vi "Load Settings from XML.vi"(8 "error in (no error)":errorcluster, 11 "Settings in":T1={"Acquisition Settings"={"AI"={"task name"="", "task_ref"="", "physical channels"="Dev1/ai0:7", "channels config"={"input terminal configuration"=0, "minimum value"=-5.0, "maximum value"=5.0}, "rate"=1000.0}, "conversions"={"ai0"={"a"=0.0, "b"=0.0}, "ai1"={"a"=0.0, "b"=0.0}, "ai2"={"a"=0.0, "b"=0.0}, "ai3"={"a"=0.0, "b"=0.0}, "ai4"={"a"=0.0, "b"=0.0}}, "compteur 0"={"task name"="CTR", "task_ref"="", "ctr"="Dev1/ctr0:3", "coeff"=4000.0}, "compteur 1"={"task name"="CTR1", "task_ref"="", "ctr"="Dev1/ctr1", "coeff"=4000.0}, "compteur 2"={"task name"="CTR2", "task_ref"="", "ctr"="Dev1/ctr2", "coeff"=4000.0}, "compteur 3"={"task name"="CTR3", "task_ref"="", "ctr"="Dev1/ctr3", "coeff"=4000.0}}, "Logging Configuration"={"Log File Base Path"=path "", "L1"={"ref"=refnum, "actif?"=FALSE, "Fsave"=0}, "L2"={"ref"=refnum, "actif?"=FALSE, "Fsave"=0}, "L3"={"ref"=refnum, "actif?"=FALSE, "Fsave"=0}, "L4"={"ref"=refnum, "actif?"=FALSE, "Fsave"=0}}, "Generation Settings"={"AO"={"task name"="AO", "task_ref"="", "physical channels"="Dev1/ao0"}, "PID"={"P"=0.0, "I"=0.0, "D"=0.0}, "conversions"={"ao0"={"a"=0.0, "b"=0.0}}, "setpoint"=0.0}, "Digital Control Configuration"={"DO"={"task name"="DO", "task_ref"="", "lines"="Dev1/port0/line2:3, Dev1/port0/line5"}}} {"Acquisition Settings"."compteur 3"."coeff" format="%0.2f"; "Acquisition Settings"."compteur 2"."coeff" format="%0.2f"; "Acquisition Settings"."compteur 1"."coeff" format="%0.2f"; "Acquisition Settings"."compteur 0"."coeff" format="%0.2f"; "Acquisition Settings"."AI"."rate" format="%0.2f"; "Acquisition Settings"."AI"."channels config"."input terminal configuration" items=["Default"=-1, "RSE"=10083, "NRSE"=10078, "Differential"=10106, "Pseudodifferential"=12529]}) -> (0 "error out":errorcluster, 3 "Settings out":T1={"Acquisition Settings"={"AI"={"task name"="", "task_ref"="", "physical channels"="Dev1/ai0:7", "channels config"={"input terminal configuration"=0, "minimum value"=-5.0, "maximum value"=5.0}, "rate"=1000.0}, "conversions"={"ai0"={"a"=0.0, "b"=0.0}, "ai1"={"a"=0.0, "b"=0.0}, "ai2"={"a"=0.0, "b"=0.0}, "ai3"={"a"=0.0, "b"=0.0}, "ai4"={"a"=0.0, "b"=0.0}}, "compteur 0"={"task name"="CTR", "task_ref"="", "ctr"="Dev1/ctr0:3", "coeff"=4000.0}, "compteur 1"={"task name"="CTR1", "task_ref"="", "ctr"="Dev1/ctr1", "coeff"=4000.0}, "compteur 2"={"task name"="CTR2", "task_ref"="", "ctr"="Dev1/ctr2", "coeff"=4000.0}, "compteur 3"={"task name"="CTR3", "task_ref"="", "ctr"="Dev1/ctr3", "coeff"=4000.0}}, "Logging Configuration"={"Log File Base Path"=path "", "L1"={"ref"=refnum, "actif?"=FALSE, "Fsave"=0}, "L2"={"ref"=refnum, "actif?"=FALSE, "Fsave"=0}, "L3"={"ref"=refnum, "actif?"=FALSE, "Fsave"=0}, "L4"={"ref"=refnum, "actif?"=FALSE, "Fsave"=0}}, "Generation Settings"={"AO"={"task name"="AO", "task_ref"="", "physical channels"="Dev1/ao0"}, "PID"={"P"=0.0, "I"=0.0, "D"=0.0}, "conversions"={"ao0"={"a"=0.0, "b"=0.0}}, "setpoint"=0.0}, "Digital Control Configuration"={"DO"={"task name"="DO", "task_ref"="", "lines"="Dev1/port0/line2:3, Dev1/port0/line5"}}} {"Acquisition Settings"."compteur 3"."coeff" format="%0.2f"; "Acquisition Settings"."compteur 2"."coeff" format="%0.2f"; "Acquisition Settings"."compteur 1"."coeff" format="%0.2f"; "Acquisition Settings"."compteur 0"."coeff" format="%0.2f"; "Acquisition Settings"."AI"."rate" format="%0.2f"; "Acquisition Settings"."AI"."channels config"."input terminal configuration" items=["Default"=-1, "RSE"=10083, "NRSE"=10078, "Differential"=10106, "Pseudodifferential"=12529]})   [LabVIEW 2014, in "PLS Settings.lvlib"]
doc: "Attempts to load previous user specified settings from an XML file.\n\nThis VI will not generate an error. If a suitable XML file can't be loaded and parsed then it will simply return the default settings."
uses:
  PLS Settings.lvlib
  Settings.ctl
  Acquisition/Hardware Configuration.ctl
  conversion.ctl
  Logging/Logging Configuration.ctl
  Generation/Hardware Configuration.ctl
  Digital Control/Hardware Configuration.ctl
  <vilib>/Utility/xml.llb/Read From XML File(string).vi
  <vilib>/Utility/xml.llb/Write to XML File(string).vi
  Acquisition/PLS Acquisition.lvlib
  Logging/PLS Logging.lvlib
  Generation/PLS Generation.lvlib
  Digital Control/PLS Digital Control.lvlib
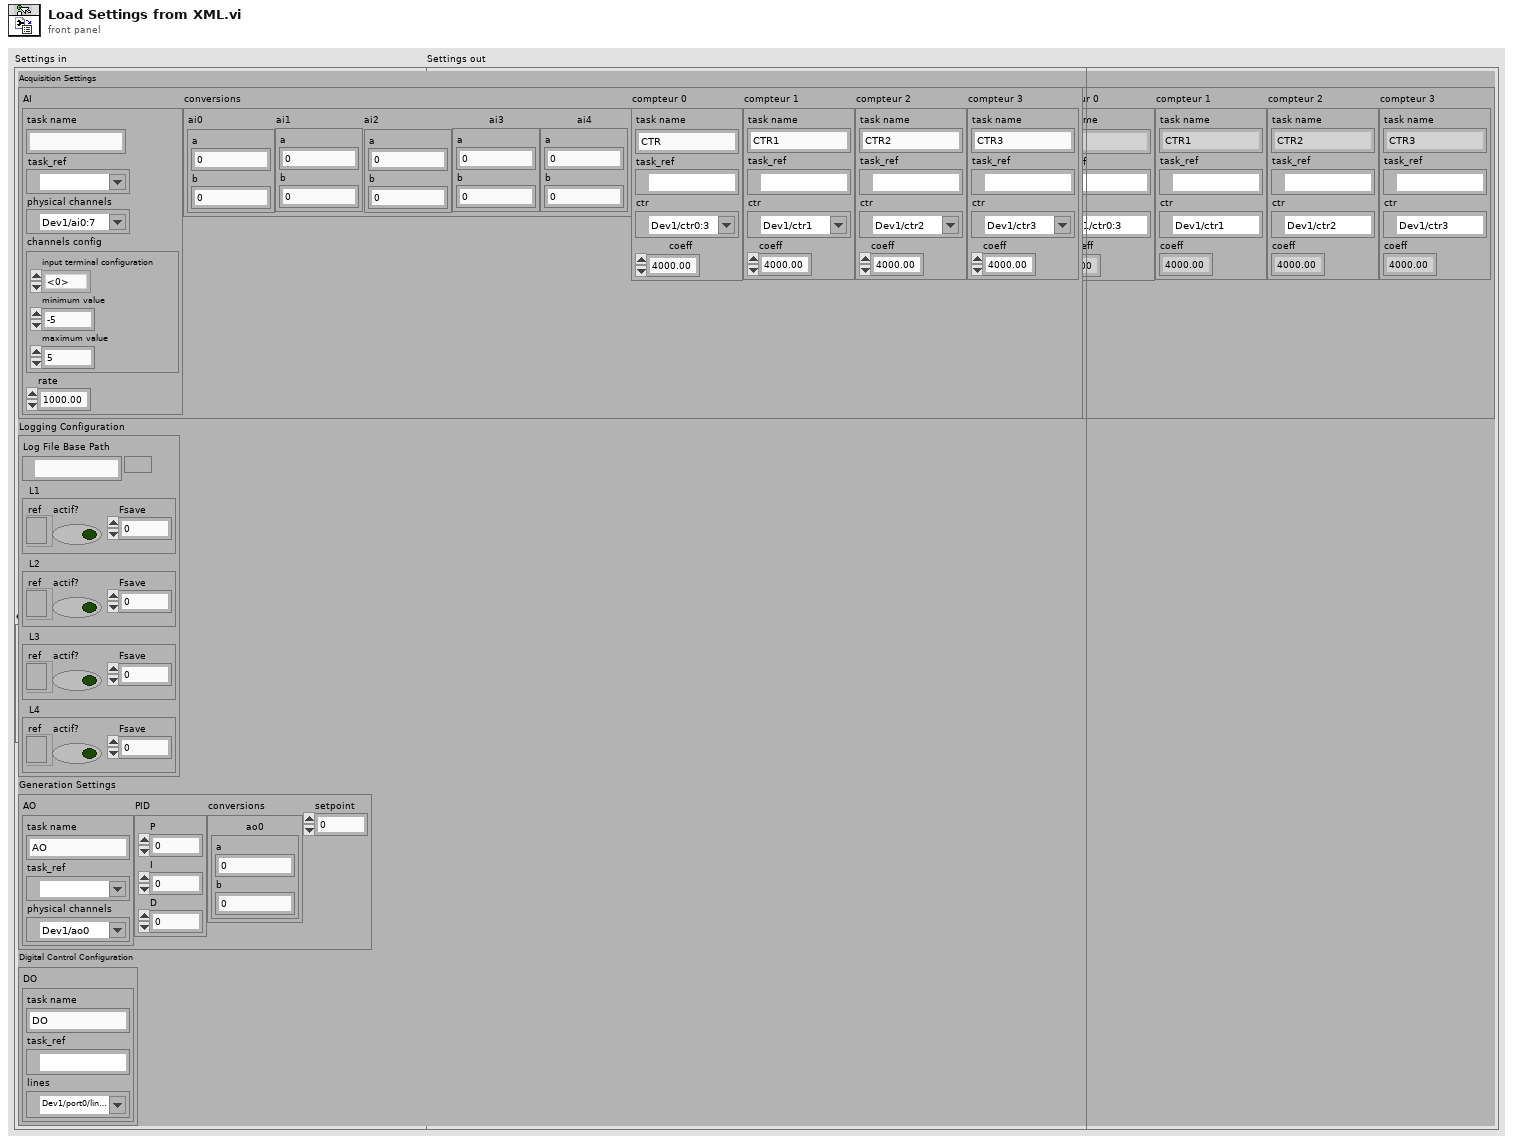
[diagram p1: front panel]
types:
  T1 = typedef "PLS Settings.lvlib/Settings.ctl" = cluster{"Acquisition Settings":T2, "Logging Configuration":T4, "Generation Settings":T5, "Digital Control Configuration":T6}
  T2 = typedef "PLS Acquisition.lvlib/Hardware Configuration.ctl" = cluster{"AI":cluster{"task name":string, "task_ref":refnum<k21>, "physical channels":tag, "channels config":cluster{"input terminal configuration":i32, "minimum value":dbl, "maximum value":dbl}, "rate":dbl}, "conversions":cluster{"ai0":T3, "ai1":T3, "ai2":T3, "ai3":T3, "ai4":T3}, "compteur 0":cluster{"task name":string, "task_ref":refnum<k21>, "ctr":tag, "coeff":dbl}, "compteur 1":cluster{"task name":string, "task_ref":refnum<k21>, "ctr":tag, "coeff":dbl}, "compteur 2":cluster{"task name":string, "task_ref":refnum<k21>, "ctr":tag, "coeff":dbl}, "compteur 3":cluster{"task name":string, "task_ref":refnum<k21>, "ctr":tag, "coeff":dbl}}
  T3 = typedef "PLS Settings.lvlib/conversion.ctl" = cluster{"a":dbl, "b":dbl}
  T4 = typedef "PLS Logging.lvlib/Logging Configuration.ctl" = cluster{"Log File Base Path":path, "L1":cluster{"ref":refnum<file>, "actif?":bool, "Fsave":i32}, "L2":cluster{"ref":refnum<file>, "actif?":bool, "Fsave":i32}, "L3":cluster{"ref":refnum<file>, "actif?":bool, "Fsave":i32}, "L4":cluster{"ref":refnum<file>, "actif?":bool, "Fsave":i32}}
  T5 = typedef "PLS Generation.lvlib/Hardware Configuration.ctl" = cluster{"AO":cluster{"task name":string, "task_ref":refnum<k21>, "physical channels":tag}, "PID":cluster{"P":dbl, "I":dbl, "D":dbl}, "conversions":cluster{"ao0":T3}, "setpoint":dbl}
  T6 = typedef "PLS Digital Control.lvlib/Hardware Configuration.ctl" = cluster{"DO":cluster{"task name":string, "task_ref":refnum<k21>, "lines":tag}}
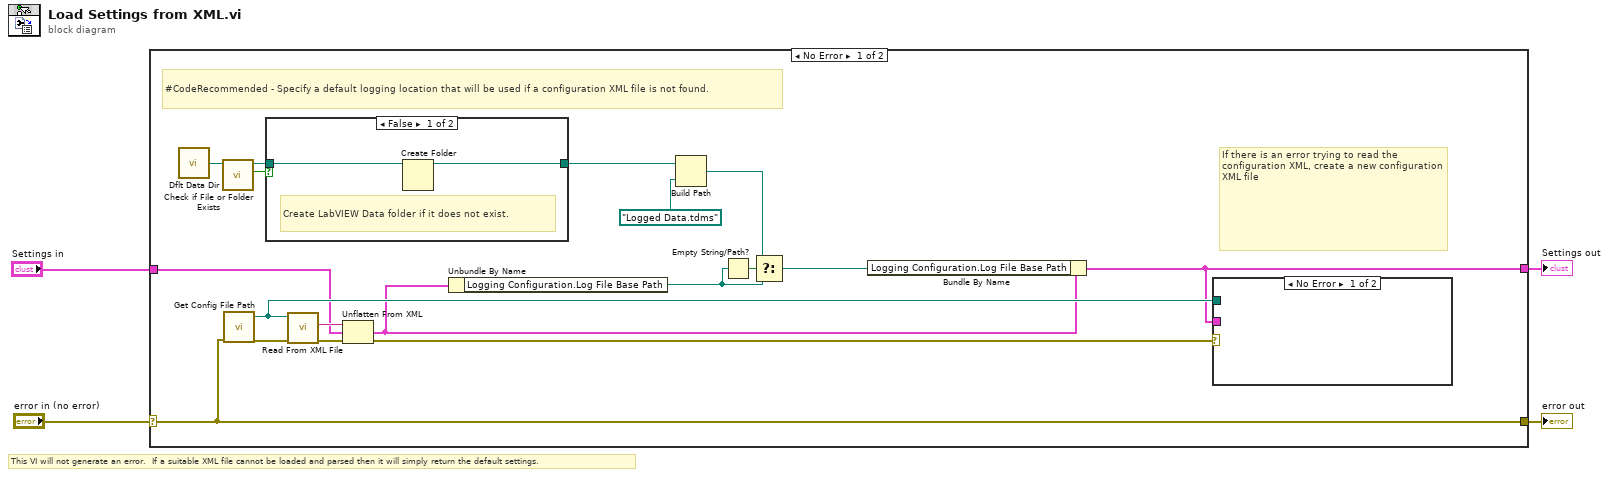
[diagram p0: block diagram]
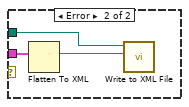
[diagram p3: hidden frame]
diagram:
  # "This VI will not generate an error.  If a suitable XML file cannot be loaded and parsed then it will simply return the default settings."
  n1 = case shown="No Error" "error in (no error)" {
    selector: "error in (no error)" -> [w20 w30]
    tunnel: [w20 w30] -> w3
    tunnel: "Settings in" -> [w15 w29]
    tunnel: [w9 w29] -> w1
    frame No Error {
      # "If there is an error trying to read the configuration XML, create a new configuration XML file"
      # "#CodeRecommended - Specify a default logging location that will be used if a configuration XML file is not found."
      n2 = call <vilib>:"Dflt Data Dir.vi"() -> ("App:Default Data Directory"=w8:path)
      n3 = call <vilib>:"Check if File or Folder Exists.vi"("path"=w8) -> ("file or folder exists?"=w7:bool, "dup path"=w6:path)  [unwired: 8 in, 1 out]
      n4 = call "Get Config File Path.vi"("error in (no error)"=w20) -> ("error out"=w22:errorcluster, "XML File Path"=w18:path)  [unwired: 9 in]
      n5 = case shown="False" w7 {
        tunnel: w6 -> [w24 w25]
        tunnel: [w23 w25] -> w5
        frame False {
          # "Create LabVIEW Data folder if it does not exist."
          n6 = Create Folder(path (use dialog)=w24) -> (created path=w23:path)  [unwired: 2 in, 2 out]
        }
        frame True {
        }
      }
      n7 = call-poly <vilib>:"Read From XML File.vi"("error in (no error)"=w22, "XML File Path"=w18) -> ("error out"=w17:errorcluster, "XML Elements"=w21:string)  [unwired: 7 in, 1 out]
      n8 = Unflatten From XML(xml string=w21, type=w15, error in (no error)=w17) -> (value=w11:T1, error out=w16:errorcluster)
      n9 = Unbundle By Name(w11) -> ("Logging Configuration.Log File Base Path"=w13:path)
      n10 = Build Path(base path=w5, name or relative path=path "Logged Data.tdms" ("App:Default Data Directory")) -> (appended path=w12:path)
      n11 = Empty String/Path?(string/path=w13) -> (empty?=w14:bool)
      n12 = Select(t=w12, s=w14, f=w13) -> (s? t:f=w10:path)
      n13 = Bundle By Name(cluster=w11, "Logging Configuration.Log File Base Path"=w10) -> (w9:T1)
      n14 = case shown="No Error" w16 {
        tunnel: w9 -> [_ w28]
        tunnel: w18 -> [_ w26]
        frame No Error {
        }
        frame Error {
          n15 = Flatten To XML(anything=w28) -> (xml string=w27:string)
          n16 = call-poly <vilib>:"Write to XML File.vi"("XML Input"=w27, "XML File Path"=w26) -> ()  [unwired: 7 in, 3 out]
        }
      }
    }
    frame Error {
    }
  }
  "error out" <- w3
  "Settings out" <- w1
